vi "Create User Event.vi"(8 "Error In":errorcluster) -> (0 "Error Out":errorcluster)   [LabVIEW 2017]
uses:
  Reference Action.ctl
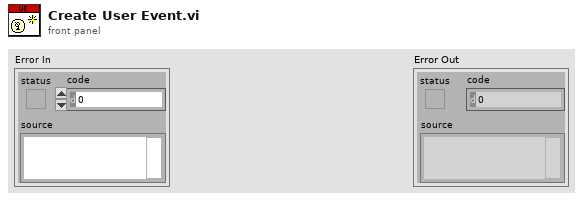
[diagram p1: front panel]
types:
  T1 = typedef "Reference Action.ctl" = enum16{"Set", "Get"}
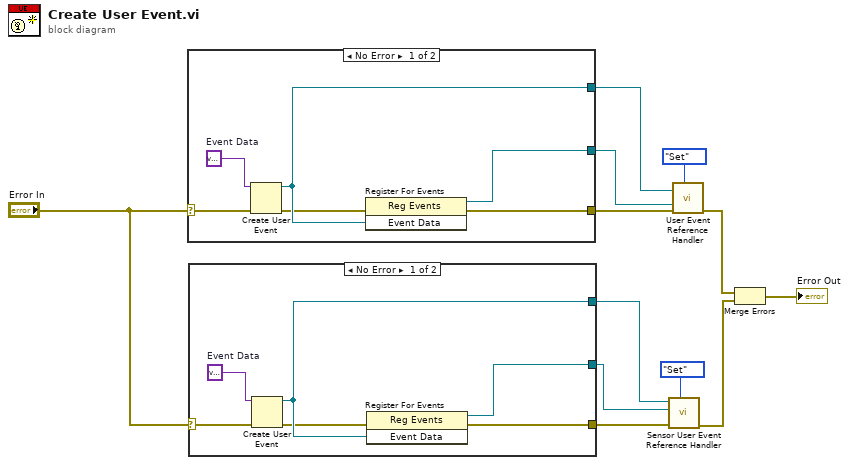
[diagram p0: block diagram]
diagram:
  n1 = case shown="No Error" "Error In" {
    selector: "Error In" -> [w14 w19]
    tunnel: [w18 _] -> w10
    tunnel: [w17 _] -> w9
    tunnel: [w15 w19] -> w12
    frame No Error {
      w13 = variant  # Event Data
      n2 = Create User Event(user event datatype=w13, error in=w14) -> (user event=w18:refnum<user-event>, error out=w16:errorcluster)
      n3 = register-events(error in=w16, w18) -> (reference out=w17:refnum<event-registration>, error out=w15:errorcluster)  [unwired: 1 in]
    }
    frame Error {
    }
  }
  n4 = case shown="No Error" "Error In" {
    selector: "Error In" -> [w21 w26]
    tunnel: [w25 _] -> w5
    tunnel: [w24 _] -> w6
    tunnel: [w22 w26] -> w7
    frame No Error {
      w20 = variant  # Event Data
      n5 = Create User Event(user event datatype=w20, error in=w21) -> (user event=w25:refnum<user-event>, error out=w23:errorcluster)
      n6 = register-events(error in=w23, w25) -> (reference out=w24:refnum<event-registration>, error out=w22:errorcluster)  [unwired: 1 in]
    }
    frame Error {
    }
  }
  n7 = call "Sensor User Event Reference Handler.vi"("Reference Action"=Reference_Action."Set", "Error In"=w7, "Event Registration Refnum In"=w6, "User Event Refnum In"=w5) -> ("Error Out"=w3:errorcluster)  [unwired: 5 in, 2 out]
  n8 = call "User Event Reference Handler.vi"("Reference Action"=Reference_Action."Set", "Error In"=w12, "Event Registration Refnum In"=w9, "User Event Refnum In"=w10) -> ("Error Out"=w2:errorcluster)  [unwired: 5 in, 2 out]
  n9 = Merge Errors(w2, w3) -> (→"Error Out":errorcluster)
